vi "Profiled_PID_TurnToAngle_Example.vi"() -> ()   [LabVIEW 2019]
uses:
  <vilib>/Rock Robotics/WPI/ThirdParty/JAS_Junk/TrajLib/ProfiledPIDController_SetPID.vi
  <vilib>/Rock Robotics/WPI/ThirdParty/JAS_Junk/TrajLib/ProfiledPIDController_SetIntegratorRange.vi
  <vilib>/Rock Robotics/WPI/ThirdParty/JAS_Junk/TrajLib/ProfiledPIDController_SetTolerance_PosVel.vi
  <vilib>/Rock Robotics/WPI/ThirdParty/JAS_Junk/TrajLib/ProfiledPIDController_DisableContInput.vi
  <vilib>/Rock Robotics/WPI/ThirdParty/JAS_Junk/TrajLib/ProfiledPIDController_EnableContInput.vi
  <vilib>/Rock Robotics/WPI/ThirdParty/JAS_Junk/TrajLib/ProfiledPIDController_Reset_PosOnly.vi
  <vilib>/Rock Robotics/WPI/ThirdParty/JAS_Junk/TrajLib/ProfiledPIDController_NewPeriod.vi
  <vilib>/Rock Robotics/WPI/ThirdParty/JAS_Junk/TrajLib/ProfiledPIDController_Calculate_Meas_Goal.vi
  <vilib>/Rock Robotics/WPI/ThirdParty/JAS_Junk/TrajLib/ProfiledPIDController_AtGoal.vi
  <vilib>/Rock Robotics/WPI/ThirdParty/JAS_Junk/TrajLib/ProfiledPIDController_AtSetpoint.vi
  <vilib>/Rock Robotics/WPI/ThirdParty/JAS_Junk/TrajLib/ProfiledPIDController_SetConstraints.vi
  <vilib>/Rock Robotics/WPI/ThirdParty/JAS_Junk/TrajLib/PIDController_GetVelocityError.vi
  <vilib>/Rock Robotics/WPI/ThirdParty/JAS_Junk/TrajLib/PIDController_GetPositionError.vi
  <vilib>/Rock Robotics/WPI/ThirdParty/JAS_Junk/TrajLib/PIDController_SetPID.vi
  <vilib>/Rock Robotics/WPI/ThirdParty/JAS_Junk/TrajLib/PIDController_SetIntegratorRange.vi
  <vilib>/Rock Robotics/WPI/ThirdParty/JAS_Junk/TrajLib/PIDController_SetTolerancePandV.vi
  <vilib>/Rock Robotics/WPI/ThirdParty/JAS_Junk/TrajLib/PIDController_DisableContinousInput.vi
  <vilib>/Rock Robotics/WPI/ThirdParty/JAS_Junk/TrajLib/PIDController_EnableContinousInput.vi
  <vilib>/Rock Robotics/WPI/ThirdParty/JAS_Junk/TrajLib/TrapProfState_New.vi
  <vilib>/Rock Robotics/WPI/ThirdParty/JAS_Junk/TrajLib/ProfiledPIDController_Reset.vi
  <vilib>/Rock Robotics/WPI/ThirdParty/JAS_Junk/TrajLib/PIDController_NewPeriod.vi
  <vilib>/Rock Robotics/SystemInterfaces/NetworkCommunication/NetComm_UsageReport_report.vi
  <vilib>/Rock Robotics/WPI/ThirdParty/JAS_Junk/TrajLib/ProfiledPIDController_SetGoal_PosOnly.vi
  <vilib>/Rock Robotics/WPI/ThirdParty/JAS_Junk/TrajLib/ProfiledPIDController_Calculate_Meas.vi
  <vilib>/Rock Robotics/WPI/ThirdParty/JAS_Junk/TrajLib/TrapProfState_Equals.vi
  <vilib>/Rock Robotics/WPI/ThirdParty/JAS_Junk/TrajLib/PIDController_AtSetpoint.vi
  <vilib>/Rock Robotics/WPI/ThirdParty/JAS_Junk/TrajLib/PIDController_Reset.vi
  <vilib>/Rock Robotics/WPI/ThirdParty/JAS_Junk/TrajLib/ProfiledPIDController_SetGoal.vi
  <vilib>/Rock Robotics/WPI/ThirdParty/JAS_Junk/TrajLib/PIDController_Calculate_SP_PV.vi
  <vilib>/Rock Robotics/WPI/ThirdParty/JAS_Junk/TrajLib/TrapProfile_New.vi
  <vilib>/Rock Robotics/WPI/ThirdParty/JAS_Junk/TrajLib/ProfiledPIDController_GetPeriod.vi
  <vilib>/Rock Robotics/WPI/ThirdParty/JAS_Junk/TrajLib/TrapProfile_Calculate.vi
  <vilib>/Rock Robotics/WPI/ThirdParty/JAS_Junk/TrajLib/ControllerUtil_GetModulusError.vi
  <vilib>/Rock Robotics/WPI/ThirdParty/JAS_Junk/TrajLib/PIDController_SetSetpoint.vi
  <vilib>/Rock Robotics/WPI/ThirdParty/JAS_Junk/TrajLib/PIDController_Calculate_PV.vi
  <vilib>/Rock Robotics/WPI/ThirdParty/JAS_Junk/TrajLib/TrapProfile_ShouldFlipAcceleration.vi
  <vilib>/Rock Robotics/WPI/ThirdParty/JAS_Junk/TrajLib/TrapProfile_Direct.vi
  <vilib>/Rock Robotics/WPI/ThirdParty/JAS_Junk/TrajLib/PIDController_GetPeriod.vi
  <vilib>/Rock Robotics/WPI/ThirdParty/JAS_Junk/TrajLib/Util_LibraryGlobals.vi
  <vilib>/Rock Robotics/WPI/ThirdParty/JAS_Junk/TrajLib/Trajectory_Library.lvlib
panel:
  in  "Tab Control":enum32{"Operation", "Tuning"}(tab)
  out "Targets along the way":T1(graph)
  in  "SP - Desired Angle\n (Deg)":dbl(slide) scale=-10.0..350.0
  out "PV - Current Angle\n (Deg)":dbl(slide) scale=-10.0..350.0
  out "Goal Chart":T2(graph)
  out "Motor Output":dbl format="%13.3f"
  out "AtSetpoint":bool
  out "AtGoal":bool
  out "PositionError  (Deg)":dbl format="%13.2f"
  out "VelocityError  (Deg/Sec)":dbl format="%13.2f"
  out "Velocity  (Deg/Sec)":dbl format="%13.2f"
  in  "Kp":dbl=0.08 format="%#_13g"
  in  "Ki":dbl=0.15 format="%#_13g"
  in  "Kd":dbl format="%#_13g"
  in  "Minimum Integral":dbl=-0.3 format="%#_13g"
  in  "Maximum Integral":dbl=0.3 format="%#_13g"
  in  "Max Speed   (Deg/Sec)":dbl=30.0 format="%#_13g"
  in  "Max Accel  (Deg/Sec^2)":dbl=5.0 format="%#_13g"
  in  "PositionTolerance\n(Deg)":dbl=1.0 format="%#_13g"
  in  "VelocityTolerance\n(Deg/Sec)":dbl=0.05 format="%#_13g"
  # "PID Tuning Parameters"
  # "Desired Profile Performance"
  # "Desired On Target Tolerance"
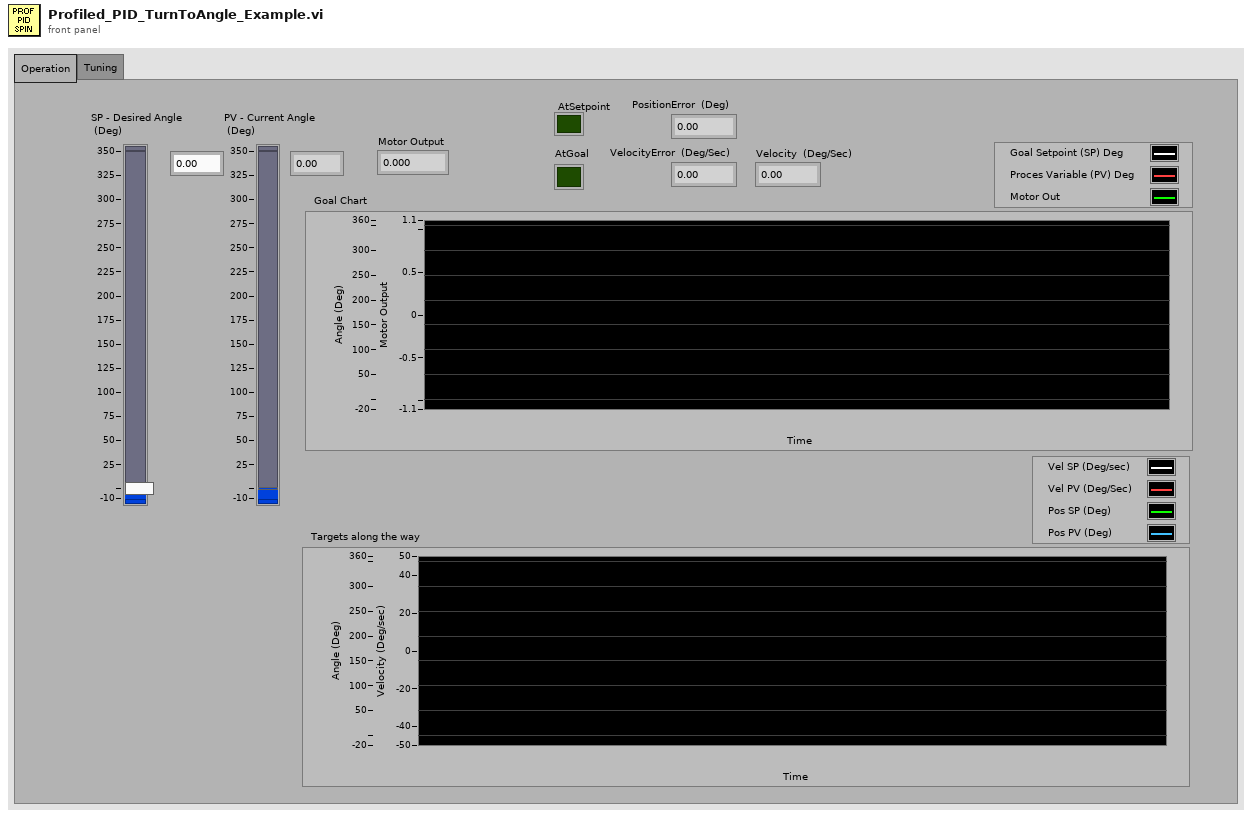
[diagram p1: front panel]
types:
  T1 = cluster{"SP - Desired Heading\n (Deg)":dbl, "PV - Current Heading\n (Deg)":dbl, "upper limit":dbl, dbl}
  T2 = cluster{"SP - Desired Position\n (Inch)":dbl, "upper limit":dbl, "upper limit":dbl}
  T3 = typedef "Trajectory_Library.lvlib/PID_ERROR_TOLERANCE.ctl" = cluster{"PositionTolerance":dbl, "VelocityTolerance":dbl}
  T4 = typedef "Trajectory_Library.lvlib/PID_TUNING.ctl" = cluster{"Kp":dbl, "Ki":dbl, "Kd":dbl, "MaximumIntegral":dbl, "MinimumIntegral":dbl}
  T5 = typedef "Trajectory_Library.lvlib/PID_INPUT_LIMITS.ctl" = cluster{"MaxInput":dbl, "MinInput":dbl, "Continuous":bool}
  T6 = typedef "Trajectory_Library.lvlib/TRAPEZOID_PROFILE_CONSTRAINT.ctl" = cluster{"MaxVelocity":dbl, "MaxAcceleration":dbl}
  T7 = typedef "Trajectory_Library.lvlib/PROFILED_PID_CONTROLLER.ctl" = cluster{"Controller":T8, "Goal":T9, "Setpoint":T9, "Constraint":T6}
  T8 = typedef "Trajectory_Library.lvlib/PID_CONTROLLER.ctl" = cluster{"Kp":dbl, "Ki":dbl, "Kd":dbl, "Period":dbl, "Max_Integral":dbl, "Min_Integral":dbl, "Max_Input":dbl, "Min_Input":dbl, "Continuous":bool, "PositionError":dbl, "VelocityError":dbl, "PrevError":dbl, "TotalError":dbl, "PositionTolerance":dbl, "VelocityTolerance":dbl, "SetPoint":dbl, "Kf":dbl, "Prev_Deriv":dbl, "Prev_Deriv 2":dbl, "DerivativeFilter":bool, "Min_Output":dbl, "Max_Output":dbl, "Prev_F_P":dbl, "Prev_F_P_2":dbl, "AntiWindupActive":bool, "Measurement":dbl}
  T9 = typedef "Trajectory_Library.lvlib/TRAPEZOID_PROFILE_STATE.ctl" = cluster{"Position":dbl, "Velocity":dbl}
  T10 = cluster{"Velocity":dbl, dbl, "Position":dbl, "modulus":dbl}
  T11 = cluster{"SP - Desired Angle\n (Deg)":dbl, "modulus":dbl, "upper limit":dbl}
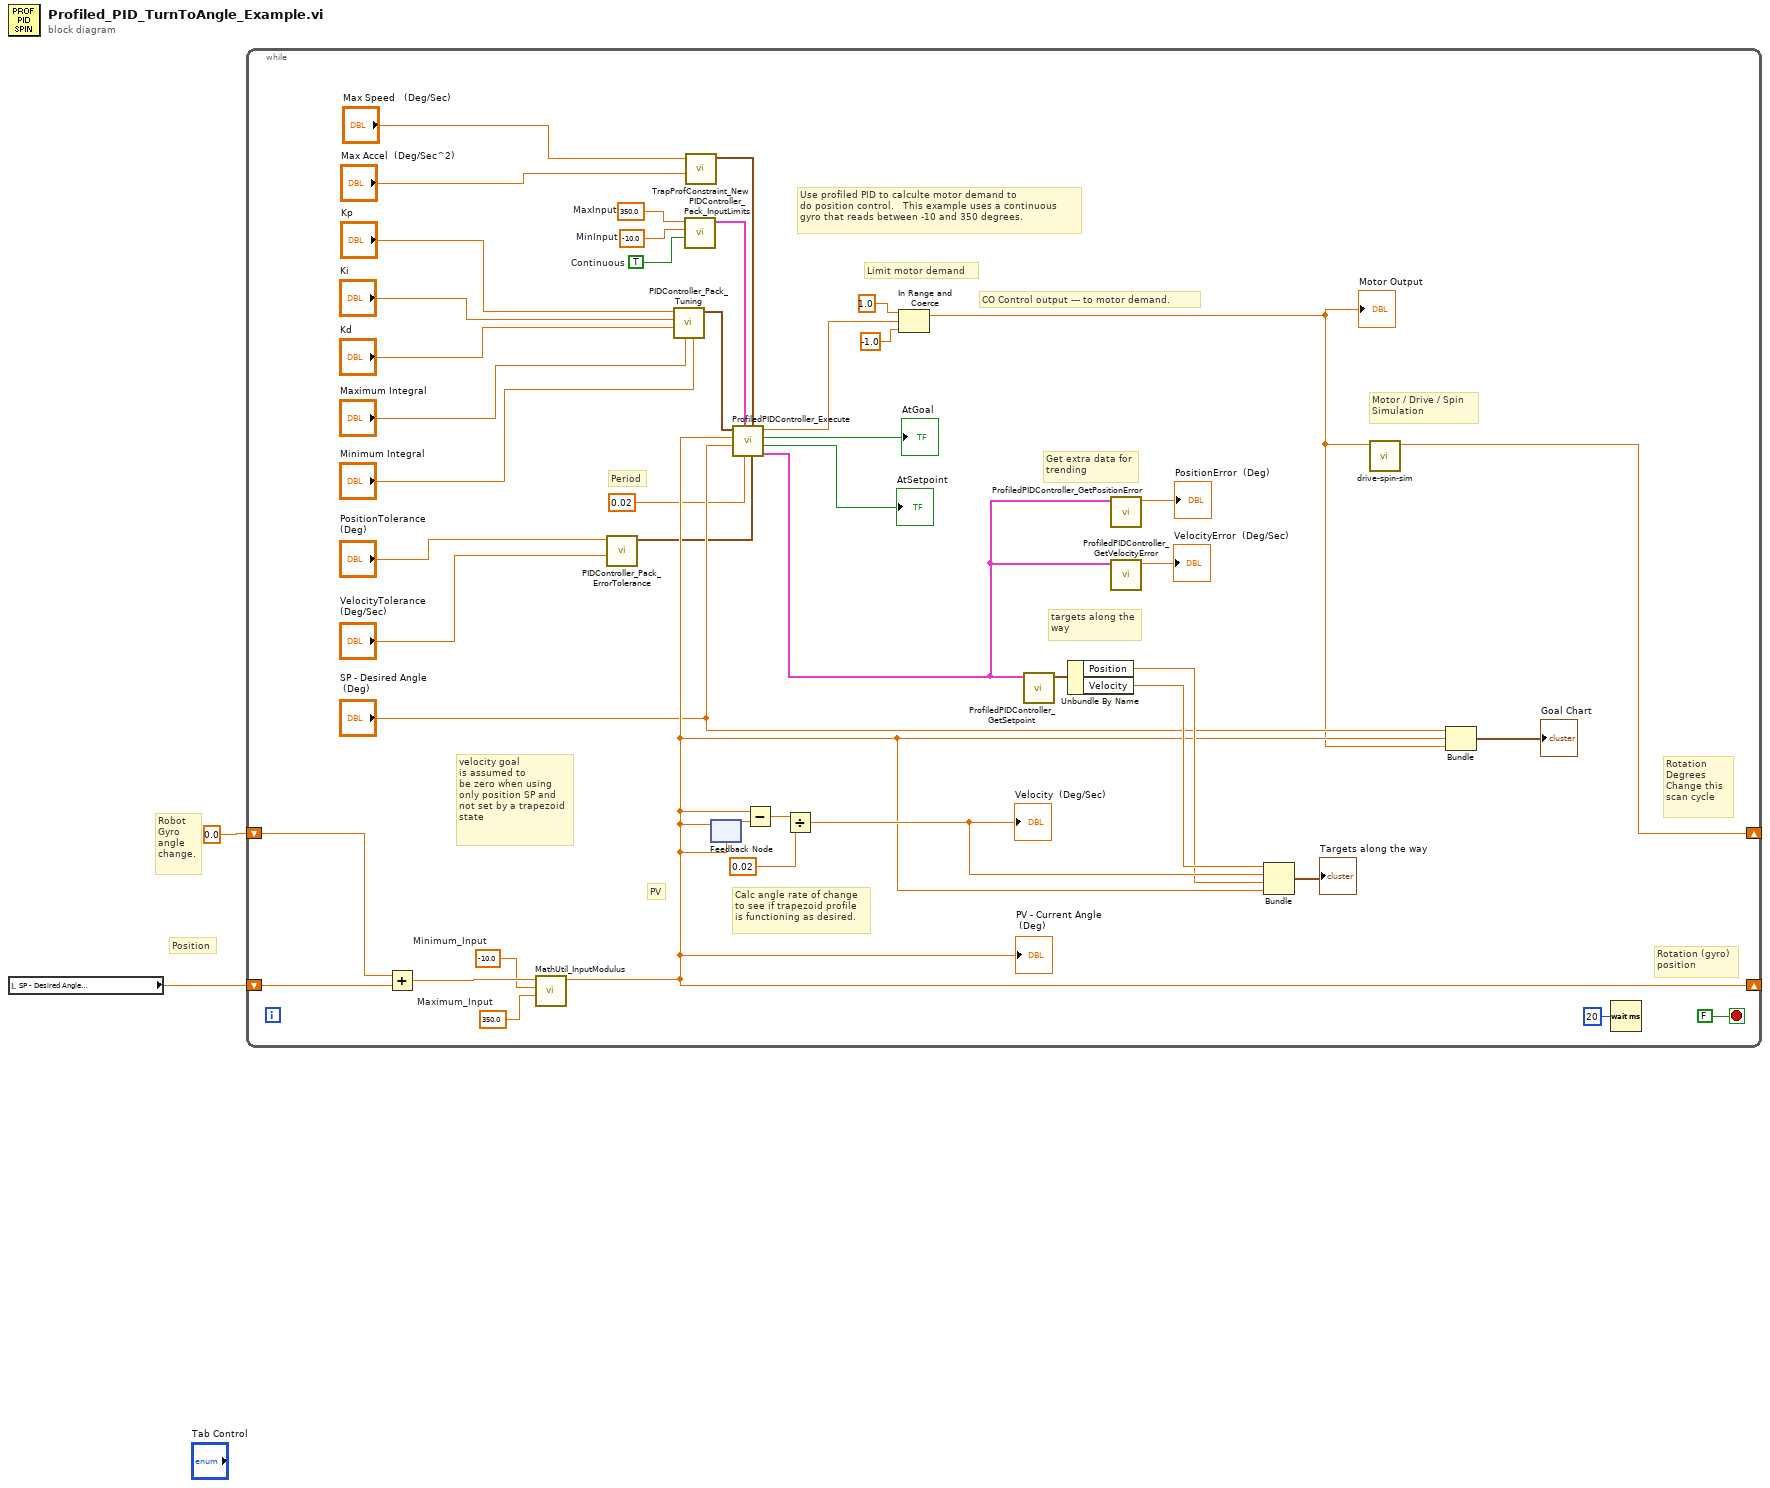
[diagram p0: block diagram]
diagram:
  # "Position"
  # "Robot\nGyro\nangle\nchange."
  n1 = local read "SP - Desired Angle\n (Deg)"() -> (w1:dbl)
  n2 = while {
    shift-right: [w22] -> _
    shift-left: w1 -> [w37]
    shift-right: [w3] -> _
    shift-left: 0.0 ("upper limit") -> [w5]
    stop <- FALSE stop-if-true
    w27 = 350.0  # MaxInput
    w26 = -10.0  # MinInput
    w25 = TRUE  # Continuous
    w29 = -10.0  # Minimum_Input
    w30 = 350.0  # Maximum_Input
    # "Use profiled PID to calculte motor demand to\ndo position control.   This example uses a continuous\ngyro that reads between -10 and 350 degrees."
    # "Rotation (gyro)\nposition"
    # "Rotation\nDegrees \nChange this \nscan cycle"
    # "CO Control output --- to motor demand."
    # "Motor / Drive / Spin\nSimulation"
    # "Get extra data for\ntrending"
    # "Period"
    # "Limit motor demand"
    # "targets along the\nway"
    # "PV"
    # "Calc angle rate of change\nto see if trapezoid profile\nis functioning as desired."
    # "velocity goal\nis assumed to \nbe zero when using\nonly position SP and\nnot set by a trapezoid\nstate"
    n3 = Add(x=w5, y=w37) -> (x+y=w31:dbl)
    n4 = call <vilib>:"MathUtil_InputModulus.vi"("Maximum_Input"=w30, "Minimum_Input"=w29, "Input"=w31) -> ("modulus"=w22:dbl)  [unwired: 8 in]
    "PV - Current Angle\n (Deg)" <- w22
    n5 = call <vilib>:"PIDController_Pack_ErrorTolerance.vi"("VelocityTolerance"="VelocityTolerance\n(Deg/Sec)", "PositionTolerance"="PositionTolerance\n(Deg)") -> ("PID Error Tolerance"=w6:T3)  [unwired: 9 in]
    n6 = call <vilib>:"PIDController_Pack_Tuning.vi"("MinimumIntegral"="Minimum Integral", "MaximumIntegral"="Maximum Integral", "Kd"="Kd", "Ki"="Ki", "Kp"="Kp") -> ("PID Tuning"=w24:T4)  [unwired: 6 in]
    n7 = call <vilib>:"PIDController_Pack_InputLimits.vi"("Continuous"=w25, "MinInput"=w26, "MaxInput"=w27) -> ("PID Input Limits"=w23:T5)  [unwired: 8 in]
    n8 = call <vilib>:"TrapProfConstraint_New.vi"("Max Accel"="Max Accel  (Deg/Sec^2)", "Max Speed (M/S)"="Max Speed   (Deg/Sec)") -> ("TRAPEZOID_PROFILE_CONSTRAINT"=w28:T6)  [unwired: 9 in]
    n9 = feedback-in #1(w22) -> ()
    n10 = feedback #1(w22) -> (w43:dbl)
    n11 = call <vilib>:"ProfiledPIDController_Execute.vi"("PID Error Tolerance"=w6, "Constraints"=w28, "Period"=0.02, "PID Input Limits"=w23, "SP-SetPoint Goal"="SP - Desired Angle\n (Deg)", "PV-Measurement"=w22, "PID Tuning"=w24) -> ("out PID_CONTROLLER"=w17:T7, "AtSetpoint"=→"AtSetpoint":bool, "AtGoal"=→"AtGoal":bool, "CO-ControlOutput"=w20:dbl)  [unwired: 1 in]
    n12 = Subtract(x=w22, y=w43) -> (x-y=w42:dbl)
    n13 = Divide(x=w42, y=0.02) -> (x/y=w33:dbl)
    "Velocity  (Deg/Sec)" <- w33
    n14 = In Range and Coerce(upper limit=1.0, x=w20, lower limit=-1.0) -> (coerced(x)=w4:dbl)  [unwired: 1 out]
    "Motor Output" <- w4
    n15 = call <vilib>:"ProfiledPIDController_GetSetpoint.vi"("in PROFILED_PID_CONTROLLER"=w17) -> ("Setpoint"=w35:T9)  [unwired: 10 in]
    n16 = Unbundle By Name(w35) -> ("Position"=w32:dbl, "Velocity"=w34:dbl)
    n17 = call <vilib>:"ProfiledPIDController_GetPositionError.vi"("in PROFILED_PID_CONTROLLER"=w17) -> ("PositionError"=→"PositionError  (Deg)":dbl)  [unwired: 10 in]
    n18 = call <vilib>:"ProfiledPIDController_GetVelocityError.vi"("in PROFILED_PID_CONTROLLER"=w17) -> ("VelocityError"=→"VelocityError  (Deg/Sec)":dbl)  [unwired: 10 in]
    n19 = Bundle("Velocity"=w34, w33, "Position"=w32, "modulus"=w22) -> (→"Targets along the way":T10)  [unwired: 1 in]
    n20 = call "drive-spin-sim.vi"("Motor Demand"=w4) -> ("Rotation Change Deg"=w3:dbl)  [unwired: 10 in]
    n21 = Bundle("SP - Desired Angle\n (Deg)"="SP - Desired Angle\n (Deg)", "modulus"=w22, "upper limit"=w4) -> (→"Goal Chart":T11)  [unwired: 1 in]
    n22 = Wait (ms)(milliseconds to wait=u32 20) -> ()  [unwired: 1 out]
  }
